vi "Main_myRIO_Helmet.vi"() -> ()   [LabVIEW 2017]
doc: "This is the myRio VI for the autonomous visor cycling (AVC) helmet. For initializing and receiving shared variables, obtaining accelerometer readings, actuating the visor and vehicle vibration warnings. By Andrew Shacker, Ning Xuan Tan, and Xander White. Spring 2018."
uses:
  <vilib>/Platform/TimedLoop/XDataNode/timing_clust.ctl
  <vilib>/Platform/TimedLoop/XDataNode/nitl_modes.ctl
  <vilib>/Platform/TimedLoop/XDataNode/wakeup.ctl
  <vilib>/myRIO/Instrument Drivers/Onboard IO/PWM/typedefs/PWM Reference.ctl
  <vilib>/myRIO/Common/Instrument Driver Framework/Utilities/typedefs/myRIO Generic Hardware Reference.ctl
  <vilib>/myRIO/Common/Instrument Driver Framework/Utilities/typedefs/Hardware Version Enum.ctl
  <vilib>/myRIO/Common/Instrument Driver Framework/Utilities/typedefs/myRIO v1.0 Reference.ctl
  <vilib>/myRIO/Common/Instrument Driver Framework/Utilities/typedefs/Generic FPGA Reference.ctl
  <vilib>/myRIO/Common/Instrument Driver Framework/myRIO v1.0/PWM/typedefs/PWM Channels Enum.ctl
  <vilib>/myRIO/Instrument Drivers/Onboard IO/PWM/typedefs/PWM Configuration.ctl
  <vilib>/userdefined/High Color/nirio_resource_hc.ctl
  <vilib>/myRIO/Instrument Drivers/Onboard IO/AI/typedefs/AI Reference.ctl
  <vilib>/myRIO/Common/Instrument Driver Framework/myRIO v1.0/AI/typedefs/AI Channels List.ctl
  <vilib>/myRIO/Common/Instrument Driver Framework/myRIO v1.0/AI/typedefs/AI Channels Enum.ctl
  <vilib>/myRIO/Common/Instrument Driver Framework/Utilities/typedefs/Analog Scaling Constants List.ctl
  <vilib>/myRIO/Common/Instrument Driver Framework/Utilities/typedefs/Analog Scaling Constants.ctl
  <vilib>/myRIO/Instrument Drivers/Onboard IO/DIO/typedefs/DIO Reference.ctl
  <vilib>/myRIO/Common/Instrument Driver Framework/myRIO v1.0/DIO/typedefs/DIO Channels List.ctl
  <vilib>/myRIO/Common/Instrument Driver Framework/myRIO v1.0/DIO/typedefs/DIO Channels Enum.ctl
  <vilib>/myRIO/Instrument Drivers/Onboard Devices/Accelerometer/typedefs/Accelerometer Reference.ctl
  <vilib>/myRIO/Common/Instrument Driver Framework/myRIO v1.0/Accelerometer/typedefs/Accelerometer Channels List.ctl
  <vilib>/myRIO/Common/Instrument Driver Framework/myRIO v1.0/Accelerometer/typedefs/Accelerometer Channels Enum.ctl
  <vilib>/myRIO/Common/Instrument Driver Framework/Utilities/vis/Is FPGA Ref Available.vi
  <vilib>/myRIO/Common/Instrument Driver Framework/myRIO v1.0/PWM/vis/myRIO v1.1 Open PWM.vi
  <vilib>/myRIO/Instrument Drivers/Onboard IO/PWM/vis/Set Duty Cycle and Frequency.vi
  <vilib>/myRIO/Common/Instrument Driver Framework/myRIO v1.0/AI/vis/myRIO v1.1 Open AI.vi
  <vilib>/myRIO/Instrument Drivers/Onboard IO/AI/vis/Read.vi
  <vilib>/myRIO/Common/Instrument Driver Framework/myRIO v1.0/DIO/vis/myRIO v1.1 Open DIO.vi
  <vilib>/myRIO/Instrument Drivers/Onboard IO/DIO/vis/Read.vi
  <vilib>/myRIO/Common/Instrument Driver Framework/myRIO v1.0/Accelerometer/vis/myRIO v1.1 Open Accelerometer.vi
  <vilib>/myRIO/Instrument Drivers/Onboard Devices/Accelerometer/vis/Read.vi
  <vilib>/myRIO/Common/Instrument Driver Framework/Utilities/vis/Validate Channels.vi
  <vilib>/myRIO/Common/Instrument Driver Framework/myRIO v1.0/PWM/vis/myRIO v1.0 Reserve PWM.vi
  <vilib>/myRIO/Common/Instrument Driver Framework/myRIO v1.0/AI/vis/myRIO v1.0 Reserve AI.vi
  <vilib>/myRIO/Common/Instrument Driver Framework/myRIO v1.0/DIO/vis/myRIO v1.0 Reserve DIO.vi
  <vilib>/myRIO/Common/Instrument Driver Framework/myRIO v1.0/Accelerometer/vis/myRIO v1.0 Reserve Accelerometer.vi
  <vilib>/myRIO/Common/Instrument Driver Framework/myRIO v1.0/UART/vis/myRIO v1.0 Close UART.vi
  <vilib>/myRIO/Common/Instrument Driver Framework/myRIO v1.0/PWM/vis/myRIO v1.0 Build MUX Configuration PWM.vi
  <vilib>/myRIO/Common/Instrument Driver Framework/myRIO v1.0/Resource Manager/vis/myRIO v1.0 Reserve Channel List.vi
  <vilib>/myRIO/Common/Instrument Driver Framework/myRIO v1.0/AI/vis/myRIO v1.0 Build MUX Configuration AI.vi
  <vilib>/myRIO/Common/Instrument Driver Framework/myRIO v1.0/DIO/vis/myRIO v1.0 Build MUX Configuration DIO.vi
  <vilib>/myRIO/Common/Instrument Driver Framework/myRIO v1.0/Accelerometer/vis/myRIO v1.0 Build MUX Configuration Accelerometer.vi
  <vilib>/myRIO/Common/Instrument Driver Framework/myRIO v1.0/Resource Manager/vis/myRIO v1.0 Create Configuration List.vi
  <vilib>/myRIO/Common/Instrument Driver Framework/myRIO v1.0/Resource Manager/vis/myRIO v1.0 Reserve Channel.vi
  <vilib>/myRIO/Common/Instrument Driver Framework/myRIO v1.0/Resource Manager/vis/myRIO v1.0 Unreserve Channel.vi
  <vilib>/myRIO/Common/Instrument Driver Framework/myRIO v1.0/Resource Manager/vis/myRIO v1.0 Build Mutex Name.vi
  duty.vi
  servostay.vi
  <vilib>/Utility/VariantDataType/GetNumericInfo.vi
  <vilib>/Utility/error.llb/Error Cluster From Error Code.vi
  <vilib>/myRIO/Common/Instrument Driver Framework/myRIO v1.0/myRIO v1.1 Open.vi
  <vilib>/myRIO/Common/Instrument Driver Framework/Utilities/vis/IO Manager.vi
  <vilib>/myRIO/Common/Instrument Driver Framework/Utilities/vis/Configuration Manager.vi
  <vilib>/myRIO/Common/Instrument Driver Framework/myRIO v1.0/Resource Manager/vis/myRIO v1.0 Configure IO.vi
  <vilib>/myRIO/Common/Instrument Driver Framework/myRIO v1.0/myRIO v1.0 Close.vi
  <vilib>/myRIO/Common/Instrument Driver Framework/myRIO v1.0/PWM/vis/myRIO v1.0 Write PWM.vi
  <vilib>/myRIO/Common/Instrument Driver Framework/myRIO v1.0/AI/vis/myRIO v1.0 Get Scaling Constants AI.vi
  <vilib>/myRIO/Common/Instrument Driver Framework/myRIO v1.0/AI/vis/myRIO v1.0 Read AI.vi
  <vilib>/myRIO/Common/Instrument Driver Framework/myRIO v1.0/DIO/vis/myRIO v1.0 Read DIO.vi
  <vilib>/myRIO/Common/Instrument Driver Framework/myRIO v1.0/Accelerometer/vis/myRIO v1.0 Get Scaling Constant Accelerometer.vi
  <vilib>/myRIO/Common/Instrument Driver Framework/myRIO v1.0/Accelerometer/vis/myRIO v1.0 Read Accelerometer.vi
  <vilib>/myRIO/Common/Instrument Driver Framework/Utilities/vis/FPGA Ref Manager.vi
  <vilib>/myRIO/Common/Instrument Driver Framework/myRIO v1.0/myRIO v1.0 Reset FPGA.vi
  <vilib>/myRIO/Common/Instrument Driver Framework/myRIO v1.0/IRQ/vis/myRIO v1.0 IRQ Info FGV.vi
  <vilib>/myRIO/Common/Instrument Driver Framework/myRIO v1.0/IRQ/vis/myRIO v1.0 Timer IRQ Info FGV.vi
  <vilib>/myRIO/Common/Instrument Driver Framework/myRIO v1.0/IRQ/vis/myRIO v1.0 ISR Agent.vi
  <vilib>/express/express arith-compare/Formula/XNode/ExpressFormulaBlockNode.xnode
  <vilib>/platform/TimedLoop/XDataNode/XDataNode.xnode
  <vilib>/myRIO/Express VI/Onboard IO/PWM/PWM Express VI.xnode
  <vilib>/myRIO/Instrument Drivers/Onboard IO/PWM/vis/myRIO PWM Open.xnode
  <vilib>/myRIO/Express VI/Onboard IO/AI/AI Express VI.xnode
  <vilib>/myRIO/Instrument Drivers/Onboard IO/AI/vis/myRIO AI Open.xnode
  <vilib>/myRIO/Express VI/Onboard Devices/Button/Button Express VI.xnode
  <vilib>/myRIO/Instrument Drivers/Onboard IO/DIO/vis/myRIO DIO Open.xnode
  <vilib>/myRIO/Express VI/Onboard Devices/Accelerometer/Accelerometer Express VI.xnode
  <vilib>/myRIO/Instrument Drivers/Onboard Devices/Accelerometer/vis/myRIO Accelerometer Open.xnode
  <vilib>/Platform/TimedLoop/XDataNode/XDNodeRunTimeDep.lvlib
  <vilib>/myRIO/Instrument Drivers/Utilities/Utilities.lvlib
  <vilib>/myRIO/Instrument Drivers/Onboard IO/PWM/PWM.lvlib
  <vilib>/myRIO/Instrument Drivers/Onboard Devices/Accelerometer/Accelerometer.lvlib
  <vilib>/myRIO/Instrument Drivers/Onboard IO/AI/AI.lvlib
  <vilib>/myRIO/Instrument Drivers/Onboard IO/DIO/DIO.lvlib
panel:
  out "Velocity Threshold":dbl
  in  "Stop":bool
  out "Accel Limits Cluster":T1
  out "Roll Rate (°/s)":dbl
  out "Pitch Rate (°/s)":dbl
  out "Pitch Angle (°)":dbl
  out "Roll Angle (°)":dbl
  out "Acceleration":T2(graph)
  # "Pitch and Roll"
  # "Acceleration"
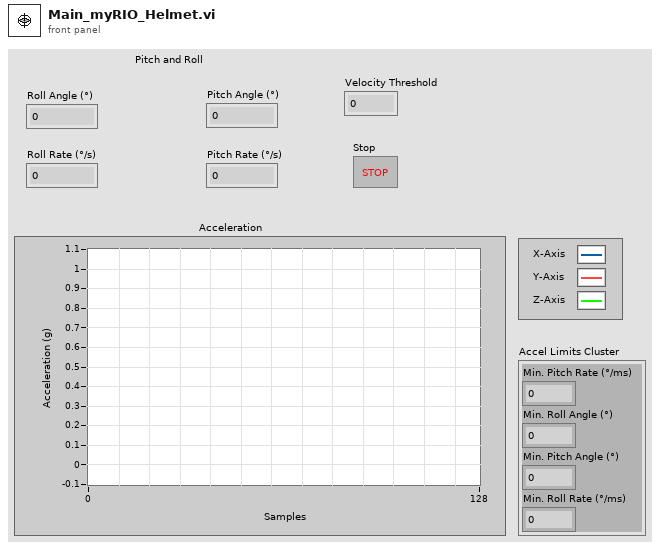
[diagram p1: front panel]
types:
  T1 = cluster{"Min. Pitch Rate (°/ms)":dbl, "Min. Roll Angle (°)":dbl, "Min. Pitch Angle (°)":dbl, "Min. Roll Rate (°/ms)":dbl}
  T2 = cluster{"X-Axis":dbl, "Y-Axis":dbl, "Z-Axis":dbl}
  T3 = typedef "PWM.lvlib/PWM Reference.ctl" = cluster{"myRIO Reference":T4, "PWM Channels Enum":T8, "PWM Configuration":T9}
  T4 = typedef "myRIO Generic Hardware Reference.ctl" = cluster{"myRIO Model":T5, "myRIO Hardware Reference":T6}
  T5 = typedef "Hardware Version Enum.ctl" = enum16{"Unknown", "myRIO-1900", "myRIO-1950", "roboRIO", "NI ELVIS RIO CM"}
  T6 = typedef "myRIO v1.0 Reference.ctl" = cluster{"Generic FPGA Reference":T7, "Allow multiple opens":bool}
  T7 = typedef "Generic FPGA Reference.ctl" = refnum<k20>
  T8 = typedef "PWM Channels Enum.ctl" = enum16{"Not Connected", "C/PWM0", "C/PWM1", "A/PWM0", "A/PWM1", "A/PWM2", "B/PWM0", "B/PWM1", "B/PWM2", "PWM/PWM0", "PWM/PWM1", "PWM/PWM2", "PWM/PWM3", "PWM/PWM4", "PWM/PWM5", "PWM/PWM6", "PWM/PWM7", "PWM/PWM8", "PWM/PWM9"}
  T9 = typedef "PWM.lvlib/PWM Configuration.ctl" = cluster{"Frequency":dbl, "Duty Cycle":dbl}
  T10 = typedef "nirio_resource_hc.ctl" = tag
  T11 = typedef "AI.lvlib/AI Reference.ctl" = cluster{"myRIO Reference":T4, "AI Channels List":T12, "AI Scaling Constants List":T14}
  T12 = typedef "AI Channels List.ctl" = T13[]
  T13 = typedef "AI Channels Enum.ctl" = enum16{"Not Connected", "AudioIn/Left", "AudioIn/Right", "C/AI0", "C/AI1", "A/AI0", "A/AI1", "A/AI2", "A/AI3", "B/AI0", "B/AI1", "B/AI2", "B/AI3", "AI/AI0", "AI/AI1", "AI/AI2", "AI/AI3"}
  T14 = typedef "Analog Scaling Constants List.ctl" = T15[]
  T15 = typedef "Analog Scaling Constants.ctl" = cluster{"LSB Weight (Volts)":dbl, "Offset (Volts)":dbl, "Signed?":bool}
  T16 = typedef "XDNodeRunTimeDep.lvlib/timing_clust.ctl" = cluster{"Expected End [f-1]":u64, "Actual End [f-1]":u64, "Finished Late? [f-1]":bool, "Expected End [i-1]":u64, "Actual End [i-1]":u64, "Finished Late? [i-1]":bool, "Expected Start [i]":u64, "Actual Start [i]":u64, "Expected Start [f]":u64, "Actual Start [f]":u64, "Source Name":string, "Structure Name":string, "Period":i64, "Deadline":i64, "Offset":i64, "Start":i64, "Priority":i32, "Timeout":i32, "Mode":T17, "Wakeup Reason":T18, "Error":errorcluster, "Source Type":string, "Secondary Source Type":string, "Global End Time":u64, "Global Start Time":u64, "Frame Duration":u64, "Iteration Duration":u64, "Assigned CPU":i32, "I/O Scan Engine Mode":u32}
  T17 = typedef "XDNodeRunTimeDep.lvlib/nitl_modes.ctl" = enum32{"No Change", "Process missed periods, maintain original phase", "Discard missed periods, maintain original phase", "Process missed periods, ignore original phase", "Discard missed periods, ignore original phase"}
  T18 = typedef "XDNodeRunTimeDep.lvlib/wakeup.ctl" = enum32{"Normal", "Aborted", "Asynchronous wakeup", "Timing source error", "Timed loop error", "Timeout"}
  T19 = typedef "DIO.lvlib/DIO Reference.ctl" = cluster{"myRIO Reference":T4, "DIO Channels List":T20}
  T20 = typedef "DIO Channels List.ctl" = T21[]
  T21 = typedef "DIO Channels Enum.ctl" = enum16{"Not Connected", "C/DIO0", "C/DIO1", "C/DIO2", "C/DIO3", "C/DIO4", "C/DIO5", "C/DIO6", "C/DIO7", "A/DIO0", "A/DIO1", "A/DIO2", "A/DIO3", "A/DIO4", "A/DIO5", "A/DIO6", "A/DIO7", "A/DIO8", "A/DIO9", "A/DIO10", "A/DIO11", "A/DIO12", "A/DIO13", "A/DIO14", "A/DIO15", "B/DIO0", "B/DIO1", "B/DIO2", "B/DIO3", "B/DIO4", "B/DIO5", "B/DIO6", "B/DIO7", "B/DIO8", "B/DIO9", "B/DIO10", "B/DIO11", "B/DIO12", "B/DIO13", "B/DIO14", "B/DIO15", "LED0", "LED1", "LED2", "LED3", "Button0", "DIO/DIO0", "DIO/DIO1", "DIO/DIO2", "DIO/DIO3", "DIO/DIO4", "DIO/DIO5", "DIO/DIO6", "DIO/DIO7", "DIO/DIO8", "DIO/DIO9", "SPI/CS0", "SPI/CS1", "SPI/CS2", "SPI/CS3", "LED RADIO (Green)", "LED RADIO (Red)", "LED COMM (Green)", "LED COMM (Red)", "LED MODE (Green)", "LED MODE (Red)"}
  T22 = typedef "Accelerometer.lvlib/Accelerometer Reference.ctl" = cluster{"myRIO Reference":T4, "Accelerometer Channels List":T23, "LSB Weight":dbl}
  T23 = typedef "Accelerometer Channels List.ctl" = T24[]
  T24 = typedef "Accelerometer Channels Enum.ctl" = enum16{"Not Connected", "X-Axis", "Y-Axis", "Z-Axis"}
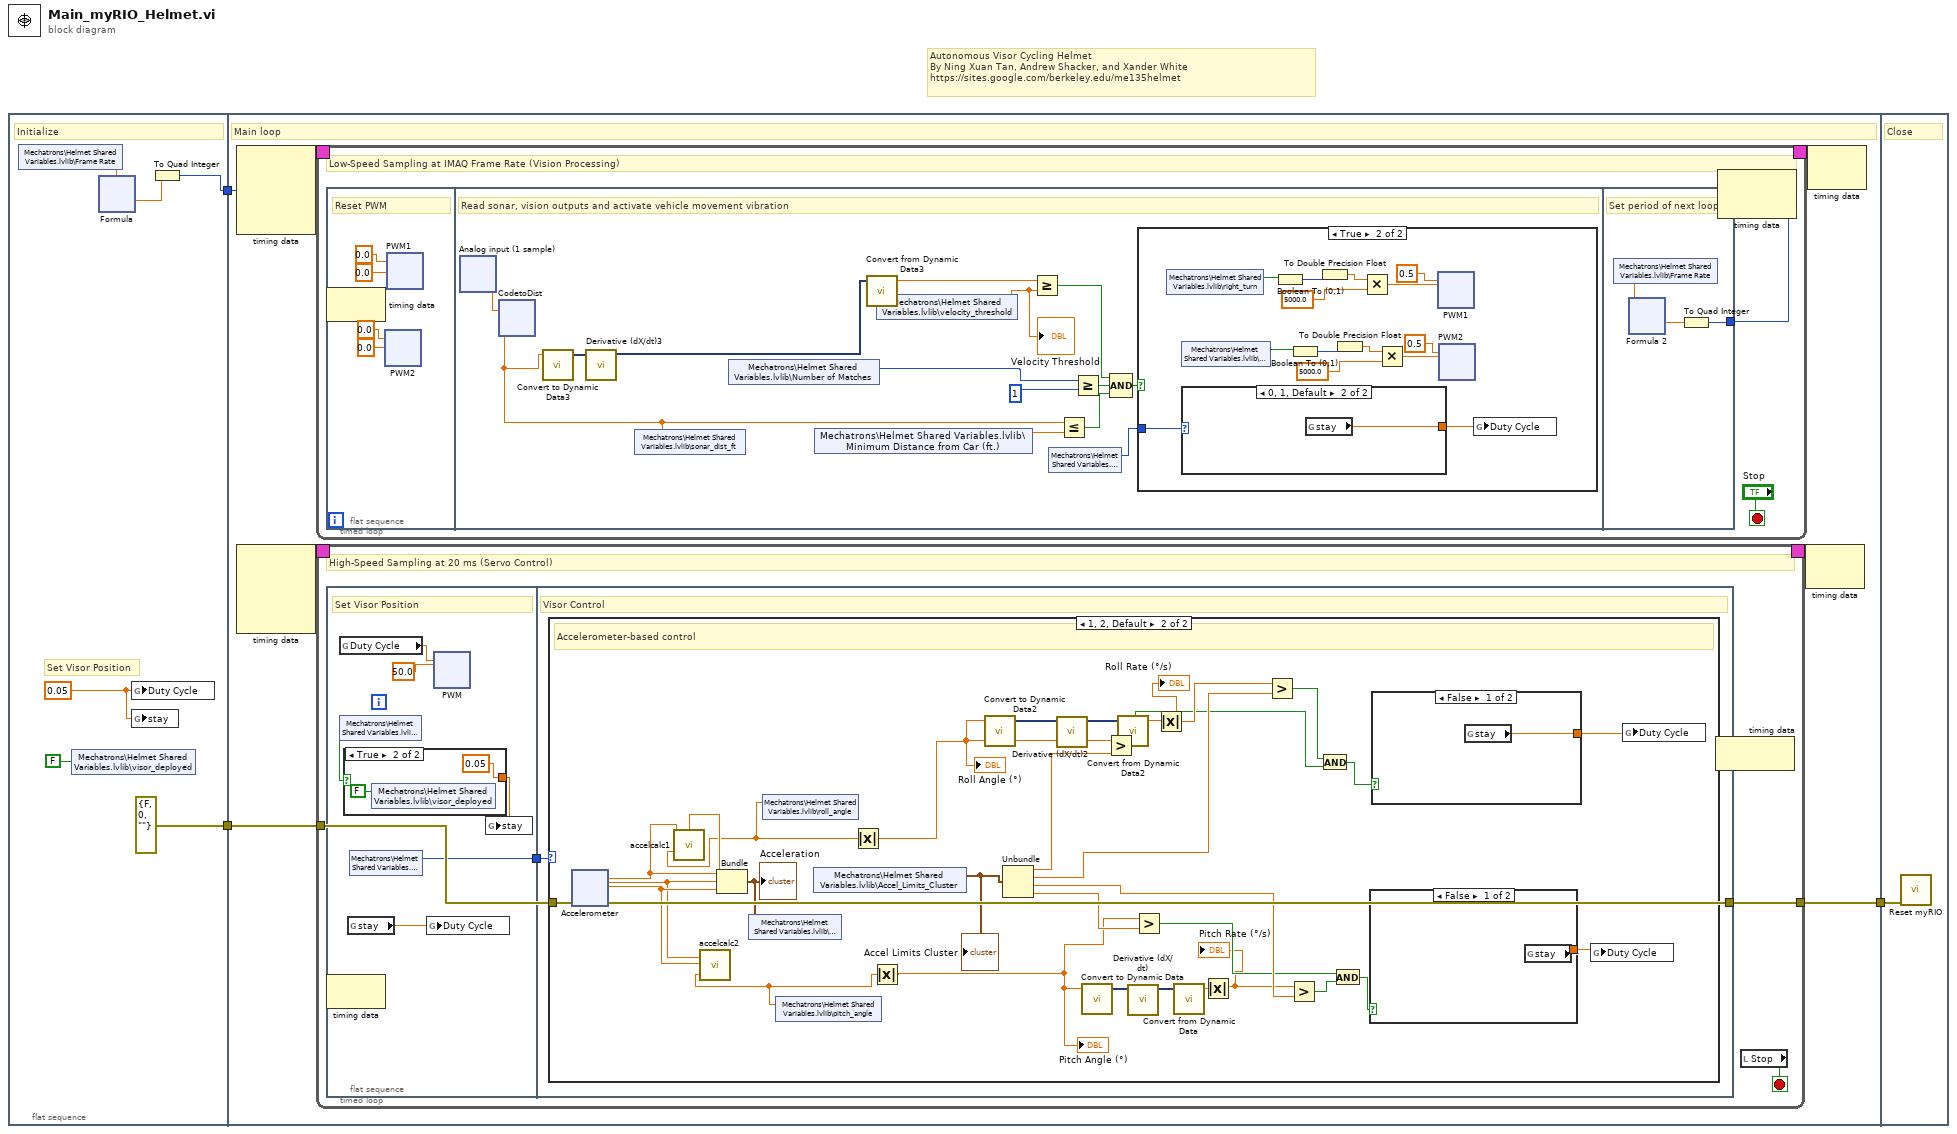
[diagram p0: block diagram]
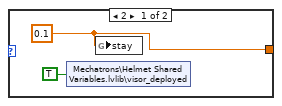
[diagram p3: hidden frame]
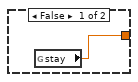
[diagram p4: hidden frame]
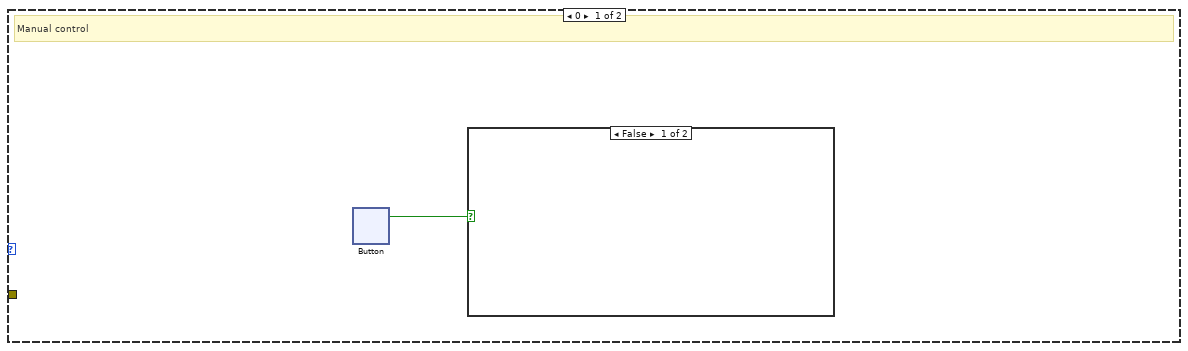
[diagram p5: hidden frame]
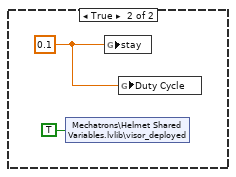
[diagram p6: hidden frame]
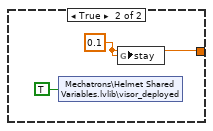
[diagram p7: hidden frame]
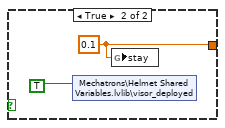
[diagram p8: hidden frame]
diagram:
  # "Autonomous Visor Cycling Helmet\nBy Ning Xuan Tan, Andrew Shacker, and Xander White\nhttps://sites.google.com/berkeley.edu/me135helmet"
  n1 = flat-sequence {
    tunnel: [errorcluster {"status"=FALSE, "code"=0, "source"=""} ("error in (no error)")] -> w3
    tunnel: [w4] -> w2
    tunnel: w3 -> [w19]
    tunnel: w2 -> [w20]
    tunnel: [w18] -> w1
    tunnel: w1 -> [w432]
    frame #0 {
      w8 = 0.05
      # "Set Visor Position"
      # "Initialize"
      n2 = shared-variable "Mechatrons\\Helmet Shared Variables.lvlib\\Frame Rate"() -> (w6:dbl)  [unwired: 1 in, 1 out]
      n3 = shared-variable "Mechatrons\\Helmet Shared Variables.lvlib\\visor_deployed"(FALSE) -> ()  [unwired: 1 in, 1 out]
      n4 = xnode ("Formula")("X1"=w6) -> ("Result"=w5:dbl)  [unwired: 1 in, 1 out]
      n5 = global write "duty.vi" "Duty Cycle"(w8) -> ()
      n6 = global write "servostay.vi" "stay"(w8) -> ()
      n7 = To Quad Integer(1:w5) -> (0:w4:i64)
    }
    frame #1 {
      # "Main loop"
      n8 = node-c288(w20) -> (w22:T16)  [unwired: 3 in]
      n9 = node-c288() -> (w24:T16)  [unwired: 4 in]
      n10 = timed-loop {
        timing: w22 -> [_]
        timing-out: [_] -> w21
        stop <- "Stop" stop-if-true
        # "Low-Speed Sampling at IMAQ Frame Rate (Vision Processing)"
        n11 = flat-sequence {
          tunnel: [w247] -> w25
          frame #0 {
            # "Reset PWM"
            n12 = xnode "PWM2"("Duty Cycle"=0.0 ("Frequency [Hz]"), "Frequency [Hz]"=0.0) -> ()  [unwired: 1 in, 1 out]
            n13 = xnode "PWM1"("Duty Cycle"=0.0 ("Frequency [Hz]"), "Frequency [Hz]"=0.0) -> ()  [unwired: 1 in, 1 out]
          }
          frame #1 {
            # "Read sonar, vision outputs and activate vehicle movement vibration"
            n14 = xnode "Analog input (1 sample)"() -> ("B/AI0 (Pin 3)"=w103:dbl)  [unwired: 1 in, 1 out]
            n15 = xnode "CodetoDist"("X"=w103) -> ("Result"=w101:dbl)  [unwired: 1 in, 1 out]
            n16 = call "Convert to Dynamic Data3"("Double"=w101) -> ("Dynamic Data Type"=w114:dynamicdata)  [unwired: 3 in]
            n17 = call "Derivative (dX/dt)3"("Signals"=w114) -> ("Result"=w113:dynamicdata)  [unwired: 5 in, 1 out]
            n18 = shared-variable "Mechatrons\\Helmet Shared Variables.lvlib\\sonar_dist_ft"(w101) -> ()  [unwired: 1 in, 1 out]
            n19 = shared-variable "Mechatrons\\Helmet Shared Variables.lvlib\\Number of Matches"() -> (w111:i32)  [unwired: 1 in, 1 out]
            n20 = shared-variable "Mechatrons\\Helmet Shared Variables.lvlib\\Minimum Distance from Car (ft.)"() -> (w109:dbl)  [unwired: 1 in, 1 out]
            n21 = call "Convert from Dynamic Data3"("Dynamic Data Type"=w113) -> ("Scalar"=w106:dbl)  [unwired: 3 in]
            n22 = shared-variable "Mechatrons\\Helmet Shared Variables.lvlib\\velocity_threshold"() -> (w102:dbl)  [unwired: 1 in, 1 out]
            "Velocity Threshold" <- w102
            n23 = Greater Or Equal?(x=w106, y=w102) -> (x >= y?=w105:bool)
            n24 = shared-variable "Mechatrons\\Helmet Shared Variables.lvlib\\Knob"() -> (w104:i32)  [unwired: 1 in, 1 out]
            n25 = Less Or Equal?(x=w101, y=w109) -> (x <= y?=w108:bool)
            n26 = Greater Or Equal?(x=w111, y=1) -> (x >= y?=w107:bool)
            n27 = Compound Arithmetic op=AND(w105, w107, w108) -> (w110:bool)
            n28 = case shown="True" w110 {
              tunnel: w104 -> [_ w120]
              frame False {
              }
              frame True {
                n29 = shared-variable "Mechatrons\\Helmet Shared Variables.lvlib\\right_turn"() -> (w128:bool)  [unwired: 1 in, 1 out]
                n30 = shared-variable "Mechatrons\\Helmet Shared Variables.lvlib\\left_turn"() -> (w124:bool)  [unwired: 1 in, 1 out]
                n31 = case shown="0, 1, Default" w120 {
                  tunnel: [w129 w131] -> w119
                  frame 2 {
                    w129 = 0.1
                    n32 = shared-variable "Mechatrons\\Helmet Shared Variables.lvlib\\visor_deployed"(TRUE) -> ()  [unwired: 1 in, 1 out]
                    n33 = global write "servostay.vi" "stay"(w129) -> ()
                  }
                  frame 0, 1, Default {
                    n34 = global read "servostay.vi" "stay"() -> (w131:dbl)
                  }
                }
                n35 = Boolean To (0,1)(Boolean=w128) -> (0, 1=w126:i16)
                n36 = Boolean To (0,1)(Boolean=w124) -> (0, 1=w122:i16)
                n37 = To Double Precision Float(number=w126) -> (double precision float=w125:dbl)
                n38 = To Double Precision Float(number=w122) -> (double precision float=w121:dbl)
                n39 = Multiply(x=w125, y=5000.0 ("Frequency [Hz]")) -> (x*y=w118:dbl)
                n40 = Multiply(x=w121, y=5000.0 ("Frequency [Hz]")) -> (x*y=w117:dbl)
                n41 = xnode "PWM1"("Duty Cycle"=0.5 ("Frequency [Hz]"), "Frequency [Hz]"=w118) -> ()  [unwired: 1 in, 1 out]
                n42 = xnode "PWM2"("Duty Cycle"=0.5 ("Frequency [Hz]"), "Frequency [Hz]"=w117) -> ()  [unwired: 1 in, 1 out]
                n43 = global write "duty.vi" "Duty Cycle"(w119) -> ()
              }
            }
          }
          frame #2 {
            # "Set period of next loop"
            n44 = shared-variable "Mechatrons\\Helmet Shared Variables.lvlib\\Frame Rate"() -> (w248:dbl)  [unwired: 1 in, 1 out]
            n45 = xnode ("Formula 2")("X1"=w248) -> ("Result"=w249:dbl)  [unwired: 1 in, 1 out]
            n46 = To Quad Integer(1:w249) -> (0:w247:i64)
          }
        }
        n47 = node-c288() -> ()  [unwired: 1 in, 1 out]
        n48 = node-c288(w25) -> ()  [unwired: 1 in, 1 out]
      }
      n49 = timed-loop "Timed Loop" {
        timing: w24 -> [_]
        timing-out: [_] -> w23
        tunnel: w19 -> [w266]
        tunnel: [w266] -> w18
        stop <- w268 stop-if-true
        # "High-Speed Sampling at 20 ms (Servo Control)"
        n50 = flat-sequence {
          tunnel: [w270] -> w267
          tunnel: w267 -> [w314]
          tunnel: w266 -> [w313]
          frame #0 {
            # "Set Visor Position"
            n51 = global read "duty.vi" "Duty Cycle"() -> (w272:dbl)
            n52 = shared-variable "Mechatrons\\Helmet Shared Variables.lvlib\\Retract"() -> (w273:bool)  [unwired: 1 in, 1 out]
            n53 = case shown="True" w273 {
              tunnel: [w275 0.05 ("stay")] -> w274
              frame False {
                n54 = global read "servostay.vi" "stay"() -> (w275:dbl)
              }
              frame True {
                n55 = shared-variable "Mechatrons\\Helmet Shared Variables.lvlib\\visor_deployed"(FALSE) -> ()  [unwired: 1 in, 1 out]
              }
            }
            n56 = global read "servostay.vi" "stay"() -> (w269:dbl)
            n57 = shared-variable "Mechatrons\\Helmet Shared Variables.lvlib\\Knob"() -> (w270:i32)  [unwired: 1 in, 1 out]
            n58 = global write "duty.vi" "Duty Cycle"(w269) -> ()
            n59 = xnode "PWM"("Duty Cycle"=w272, "Frequency [Hz]"=50.0 ("Frequency")) -> ()  [unwired: 1 in, 1 out]
            n60 = global write "servostay.vi" "stay"(w274) -> ()
          }
          frame #1 {
            # "Visor Control"
            n61 = case shown="1, 2, Default" w314 {
              tunnel: w313 -> [_ w363]
              frame 0 {
                # "Manual control"
                n62 = xnode "Button"() -> ("Value"=w315:bool)  [unwired: 1 in, 1 out]
                n63 = case shown="False" w315 {
                  frame False {
                  }
                  frame True {
                    w317 = 0.1
                    n64 = shared-variable "Mechatrons\\Helmet Shared Variables.lvlib\\visor_deployed"(TRUE) -> ()  [unwired: 1 in, 1 out]
                    n65 = global write "servostay.vi" "stay"(w317) -> ()
                    n66 = global write "duty.vi" "Duty Cycle"(w317) -> ()
                  }
                }
              }
              frame 1, 2, Default {
                # "Accelerometer-based control"
                n67 = xnode "Accelerometer"("error in (no error)"=w363) -> ("X-Axis"=w376:dbl, "Y-Axis"=w374:dbl, "Z-Axis"=w375:dbl)  [unwired: 1 out]
                n68 = call "accelcalc1.vi"("X"=w376, "Z"=w375) -> ("Result"=w355:dbl)  [unwired: 12 in, 1 out]
                n69 = call "accelcalc2.vi"("Y"=w374, "Z"=w375) -> ("Result"=w353:dbl)  [unwired: 12 in, 1 out]
                n70 = Bundle("X-Axis"=w376, "Y-Axis"=w374, "Z-Axis"=w375) -> (w364:T2)  [unwired: 1 in]
                "Acceleration" <- w364
                n71 = shared-variable "Mechatrons\\Helmet Shared Variables.lvlib\\xyz_accel"(w364) -> ()  [unwired: 1 in, 1 out]
                n72 = shared-variable "Mechatrons\\Helmet Shared Variables.lvlib\\roll_angle"(w355) -> ()  [unwired: 1 in, 1 out]
                n73 = shared-variable "Mechatrons\\Helmet Shared Variables.lvlib\\pitch_angle"(w353) -> ()  [unwired: 1 in, 1 out]
                n74 = shared-variable "Mechatrons\\Helmet Shared Variables.lvlib\\Accel_Limits_Cluster"() -> (w377:T1)  [unwired: 1 in, 1 out]
                "Accel Limits Cluster" <- w377
                n75 = Absolute Value(x=w355) -> (abs(x)=w356:dbl)
                "Roll Angle (°)" <- w356
                n76 = Absolute Value(x=w353) -> (abs(x)=w354:dbl)
                "Pitch Angle (°)" <- w354
                n77 = call "Convert to Dynamic Data2"("Double"=w356) -> ("Dynamic Data Type"=w371:dynamicdata)  [unwired: 3 in]
                n78 = Unbundle(w377) -> ("Min. Pitch Rate (°/ms)"=w381:dbl, "Min. Roll Angle (°)"=w378:dbl, "Min. Pitch Angle (°)"=w379:dbl, "Min. Roll Rate (°/ms)"=w380:dbl)
                n79 = call "Derivative (dX/dt)2"("Signals"=w371) -> ("Result"=w382:dynamicdata)  [unwired: 5 in, 1 out]
                n80 = call "Convert to Dynamic Data"("Double"=w354) -> ("Dynamic Data Type"=w369:dynamicdata)  [unwired: 3 in]
                n81 = Greater?(x=w356, y=w381) -> (0:w357:bool)
                n82 = call "Convert from Dynamic Data2"("Dynamic Data Type"=w382) -> ("Scalar"=w361:dbl)  [unwired: 3 in]
                n83 = call "Derivative (dX/dt)"("Signals"=w369) -> ("Result"=w368:dynamicdata)  [unwired: 5 in, 1 out]
                n84 = Greater?(x=w354, y=w380) -> (0:w365:bool)
                n85 = Absolute Value(x=w361) -> (abs(x)=w362:dbl)
                "Roll Rate (°/s)" <- w362
                n86 = call "Convert from Dynamic Data"("Dynamic Data Type"=w368) -> ("Scalar"=w359:dbl)  [unwired: 3 in]
                n87 = Absolute Value(x=w359) -> (abs(x)=w360:dbl)
                "Pitch Rate (°/s)" <- w360
                n88 = Greater?(x=w362, y=w378) -> (0:w358:bool)
                n89 = Greater?(x=w360, y=w379) -> (0:w366:bool)
                n90 = And(x=w358, y=w357) -> (x .and. y?=w373:bool)
                n91 = And(x=w365, y=w366) -> (x .and. y?=w367:bool)
                n92 = case shown="False" w367 {
                  tunnel: [w386 w388] -> w370
                  frame False {
                    n93 = global read "servostay.vi" "stay"() -> (w386:dbl)
                  }
                  frame True {
                    w388 = 0.1
                    n94 = shared-variable "Mechatrons\\Helmet Shared Variables.lvlib\\visor_deployed"(TRUE) -> ()  [unwired: 1 in, 1 out]
                    n95 = global write "servostay.vi" "stay"(w388) -> ()
                  }
                }
                n96 = case shown="False" w373 {
                  tunnel: [w383 w385] -> w372
                  frame False {
                    n97 = global read "servostay.vi" "stay"() -> (w383:dbl)
                  }
                  frame True {
                    w385 = 0.1
                    n98 = shared-variable "Mechatrons\\Helmet Shared Variables.lvlib\\visor_deployed"(TRUE) -> ()  [unwired: 1 in, 1 out]
                    n99 = global write "servostay.vi" "stay"(w385) -> ()
                  }
                }
                n100 = global write "duty.vi" "Duty Cycle"(w370) -> ()
                n101 = global write "duty.vi" "Duty Cycle"(w372) -> ()
              }
            }
          }
        }
        n102 = node-c288() -> ()  [unwired: 1 in, 1 out]
        n103 = node-c288() -> ()  [unwired: 1 in, 1 out]
        n104 = local read "Stop"() -> (w268:bool)
      }
      n105 = node-c288(w23) -> ()  [unwired: 1 out]
      n106 = node-c288(w21) -> ()  [unwired: 1 out]
    }
    frame #2 {
      # "Close"
      n107 = call <vilib>:"Reset myRIO.vi"("error in (no error)"=w432) -> ()  [unwired: 10 in, 1 out]
    }
  }
